vi "leexel.vi"(5 "path":string) -> (1 "array 5":string[][](array[string]))   [LabVIEW 2012]
panel:
  in  "array 4":string[][](array[string])
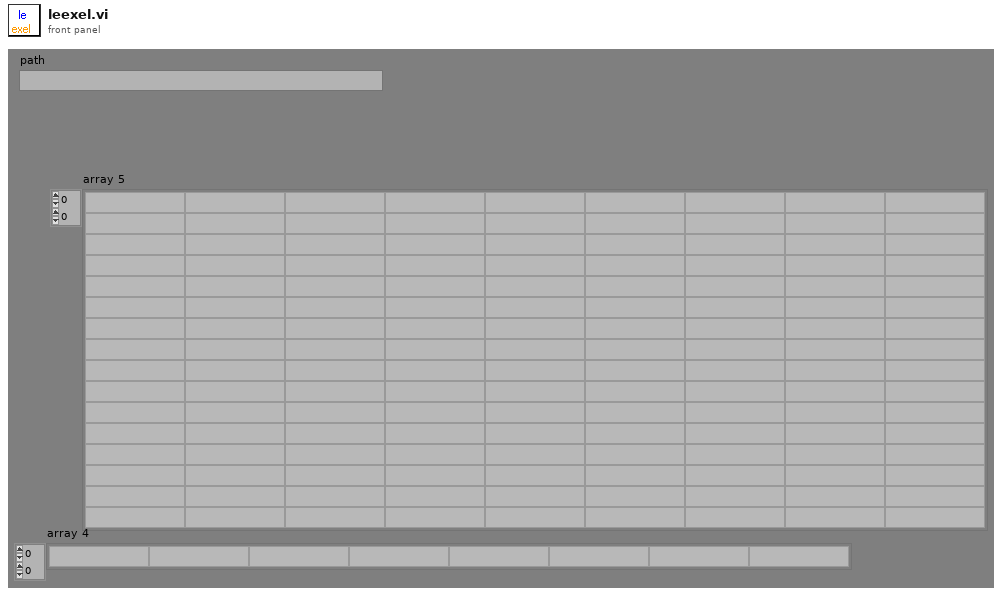
[diagram p1: front panel]
types:
  T1 = enum16{"open", "open or create", "create or replace", "create"}
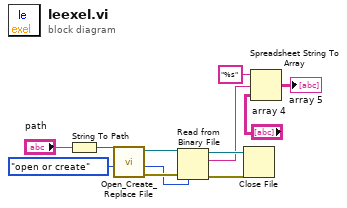
[diagram p0: block diagram]
diagram:
  n1 = String To Path(string="path") -> (path=w11:path)
  n2 = call <vilib>:"Open_Create_Replace File.vi"("function (open:0)"=T1."open or create", "file path"=w11) -> ("error out"=w9:errorcluster, "file size (bytes)"=w8:i32, "refnum"=w5:refnum<file>)  [unwired: 6 in, 1 out]
  n3 = Read from Binary File(8:w9, 10:w8, 11:w5) -> (0:w7:errorcluster, 2:w3:string, 3:w6:refnum<file>)  [unwired: 3 in, 1 out]
  n4 = Close File(refnum=w6, error in=w7) -> ()  [unwired: 2 out]
  n5 = Spreadsheet String To Array(format string="%s", spreadsheet string=w3, array type (2D Dbl)="array 4") -> (array=→"array 5":string[][])  [unwired: 1 in]
